vi "Intake Global.vi"() -> ()   [LabVIEW 2019]
uses:
  Intake Mode Type Def.ctl
  <vilib>/Rock Robotics/WPI/Solenoid/WPI_SolenoidValue.ctl
  Intake Command Type Def.ctl
panel:
  in  "Intake Command":T1
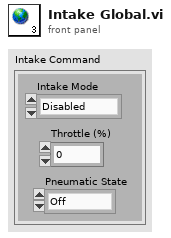
[diagram p1: front panel]
types:
  T1 = typedef "Intake Command Type Def.ctl" = cluster{"Intake Mode":T2, "Throttle (%)":dbl, "Pneumatic State":T3}
  T2 = typedef "Intake Mode Type Def.ctl" = enum16{"Disabled", "Enabled"}
  T3 = typedef "WPI_SolenoidValue.ctl" = enum16{"Off", "On", "Forward", "Reverse"}
diagram:
